vi "FdxQueryResourceCvi.vi"(8 "error in":errorcluster, 9 "ResourceType":u32(ring) items=["Board", "Port"], 10 "SrvName":string="local", 11 "ResourceID":u32) -> (0 "error out":errorcluster, 1 "ResourceInfo":T1 {"PortMode" items=[" FDX_SINGLE", "FDX_REDUNDANT"]}, 3 "ResourceID out":u32)   [LabVIEW 2020, in "AIM664LV.lvlib"]
doc: "To get information about one resource which clients are using this resource."
uses:
  AIM664LV.lvlib
  FdxGlobalDllPath.vi
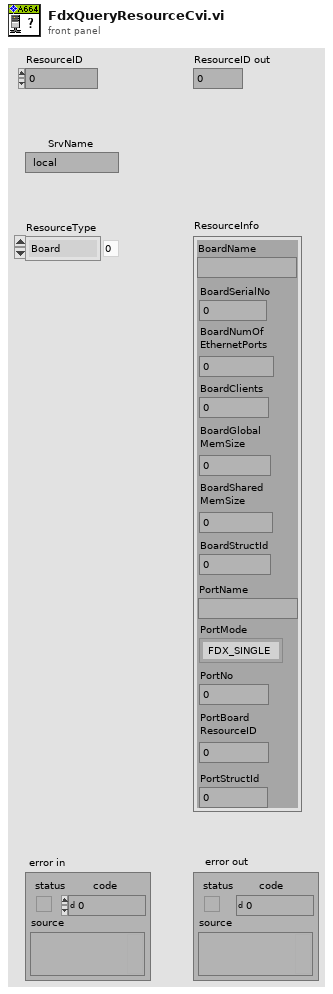
[diagram p1: front panel]
types:
  T1 = cluster{"BoardName":string, "BoardSerialNo":u32, "BoardNumOf\nEthernetPorts":u32, "BoardClients":u32, "BoardGlobal\nMemSize":u32, "BoardShared\nMemSize":u32, "BoardStructId":u32, "PortName":string, "PortMode":u32, "PortNo":u32, "PortBoard\nResourceID":u32, "PortStructId":u32}
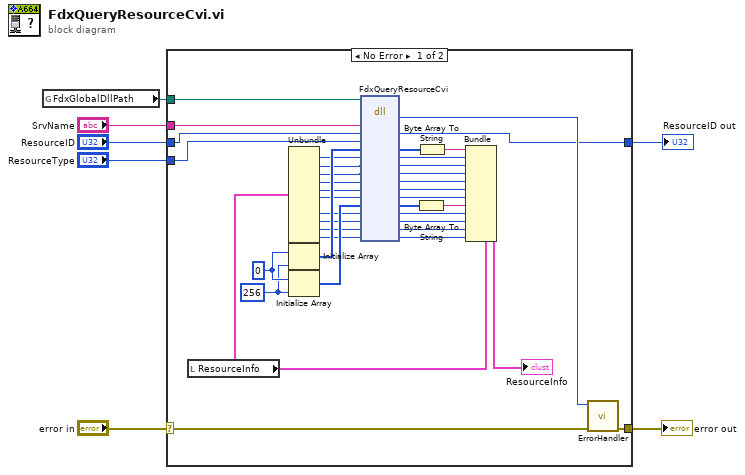
[diagram p0: block diagram]
diagram:
  n1 = global read "FdxGlobalDllPath.vi" "FdxGlobalDllPath"() -> (w5:path)
  n2 = case shown="No Error" "error in" {
    selector: "error in" -> [w44 w47]
    tunnel: [w45 w47] -> w7
    tunnel: w5 -> [w12 _]
    tunnel: "SrvName" -> [w11 _]
    tunnel: "ResourceID" -> [w10 w46]
    tunnel: "ResourceType" -> [w9 _]
    tunnel: [w8 w46] -> w1
    frame No Error {
      w35 = u8 0 ("element")
      w34 = 256 ("dimension size")
      n3 = local read "ResourceInfo"() -> (w13:T1)
      n4 = Unbundle(w13) -> ("BoardSerialNo"=w23:u32, "BoardNumOf\nEthernetPorts"=w22:u32, "BoardClients"=w21:u32, "BoardGlobal\nMemSize"=w20:u32, "BoardShared\nMemSize"=w19:u32, "BoardStructId"=w18:u32, "PortMode"=w17:u32, "PortNo"=w16:u32, "PortBoard\nResourceID"=w14:u32, "PortStructId"=w15:u32)  [unwired: 2 out]
      n5 = Initialize Array(w35, w34) -> (w33:u8[])
      n6 = Initialize Array(w35, w34) -> (w36:u8[])
      n7 = dll-call lib="aim_fdx.19.dll" fn="FdxQueryResourceCvi"(path in=w12, "SrvName"=w11, "ResourceID"=w10, "ResourceType"=w9, "BoardName"=w33, "BoardSerialNo"=w23, "BoardNumOfEthernetPorts"=w22, "BoardClients"=w21, "BoardGlobalMemSize"=w20, "BoardSharedMemSize"=w19, "BoardStructId"=w18, "PortName"=w36, "PortMode"=w17, "PortNo"=w16, "PortBoardResourceID"=w14, "PortStructId"=w15) -> ("status"=w43:i32, "ResourceID"=w8:u32, "BoardName"=w32:u8[], "BoardSerialNo"=w42:u32, "BoardNumOfEthernetPorts"=w41:u32, "BoardClients"=w40:u32, "BoardGlobalMemSize"=w39:u32, "BoardSharedMemSize"=w38:u32, "BoardStructId"=w37:u32, "PortName"=w30:u8[], "PortMode"=w28:u32, "PortNo"=w27:u32, "PortBoardResourceID"=w26:u32, "PortStructId"=w25:u32)  [unwired: 3 in, 3 out]
      n8 = Byte Array To String(unsigned byte array=w30) -> (string=w29:string)
      n9 = Byte Array To String(unsigned byte array=w32) -> (string=w31:string)
      n10 = Bundle(cluster=w13, "BoardName"=w31, "BoardSerialNo"=w42, "BoardNumOf\nEthernetPorts"=w41, "BoardClients"=w40, "BoardGlobal\nMemSize"=w39, "BoardShared\nMemSize"=w38, "BoardStructId"=w37, "PortName"=w29, "PortMode"=w28, "PortNo"=w27, "PortBoard\nResourceID"=w26, "PortStructId"=w25) -> (→"ResourceInfo":T1)
      n11 = call "ErrorHandler.vi"("error in"=w44, "AIM Error"=w43) -> ("error out"=w45:errorcluster)  [unwired: 9 in]
    }
    frame Error {
    }
  }
  "error out" <- w7
  "ResourceID out" <- w1
